vi "Main.vi"() -> (0 "queue":refnum<queue>)   [LabVIEW 2012]
uses:
  <vilib>/gmath/statdist.llb/Uniform Random.vi
  <vilib>/gmath/NI_Gmath.lvlib
panel:
  in  "Boolean":bool
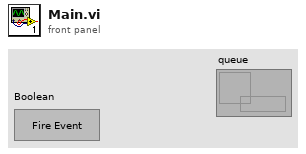
[diagram p1: front panel]
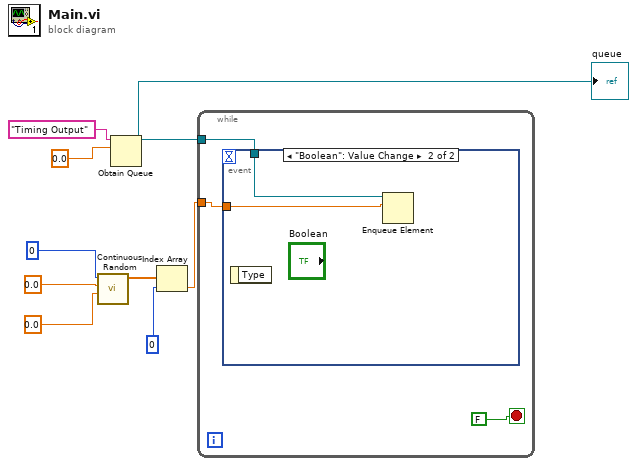
[diagram p0: block diagram]
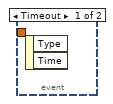
[diagram p2: hidden frame]
diagram:
  n1 = call-poly <vilib>:"Continuous Random.vi"("xmax"=0.0, "xmin"=0.0, "samples"=0) -> ("uniform random data"=w4:dbl[])  [unwired: 7 in, 1 out]
  n2 = Obtain Queue(name (unnamed)="Timing Output", element data type=0.0) -> (queue out=w1:refnum<queue>)  [unwired: 3 in, 2 out]
  "queue" <- w1
  n3 = Index Array(array=w4, index=0) -> (element=w3:dbl)
  n4 = while {
    tunnel: w1 -> [w12]
    tunnel: w3 -> [w11]
    stop <- FALSE stop-if-true
    n5 = event shown="[1] \"Boolean\": Value Change" {
      selector: _ -> [_ _]
      dyn-events: _ -> [_ _]
      timeout: _ -> [_ _]
      tunnel: w12 -> [_ w14]
      tunnel: w11 -> [_ w13]
      event Timeout {
        n6 = event-data() -> ()  [unwired: 1 in, 2 out]
      }
      event "Boolean": Value Change {
        n7 = event-data() -> ()  [unwired: 1 in, 1 out]
        n8 = Enqueue Element(queue=w14, element=w13) -> ()  [unwired: 2 in, 3 out]
      }
    }
  }
